vi "Find All Zeros of f(x) (Formula).vi"(6 "formula":string, 7 "accuracy":dbl=1e-08 format="%.2e", 8 "end":dbl=1.0 format="%.2f", 9 "start":dbl format="%.2f", 10 "algorithm":u16(ring) items=["Ridders", "Newton Raphson"], 11 "step type":u16(ring) items=["fixed function", "modified function"]) -> (0 "error":i32, 1 "ticks":u32, 2 "f(Zeros)":dbl[](array[numeric]) format="%.2f", 3 "Zeros":dbl[](array[numeric]) format="%.2f")   [LabVIEW 2014, in "NI_Gmath.lvlib"]
doc: "Determines all zeros of a 1D function in a given interval. You must manually select the polymorphic instance to use."
uses:
  NI_Gmath.lvlib
panel:
  # "Example:\n\n accuracy: 1E-8 \n step type: fixed function \n algorithm: Ridders \n start: 0.0\n end: 1.0\n formula: x^2+sin(x)-1"
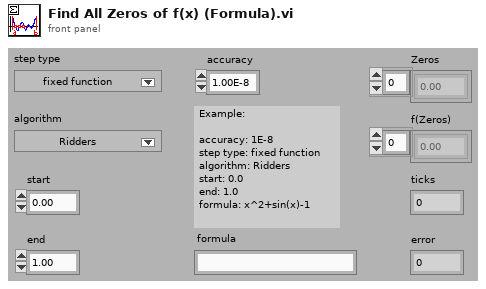
[diagram p1: front panel]
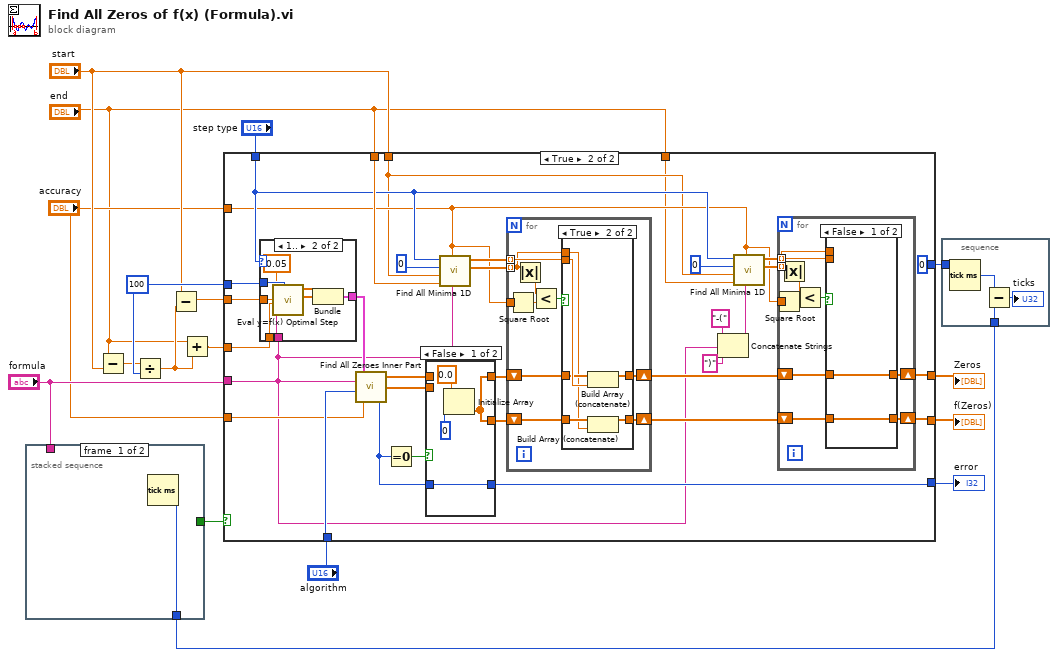
[diagram p0: block diagram]
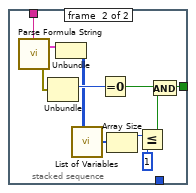
[diagram p2: hidden frame]
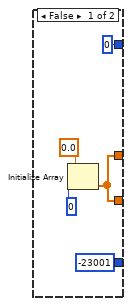
[diagram p3: hidden frame]
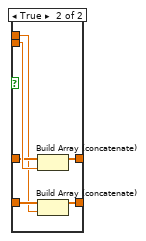
[diagram p4: hidden frame]
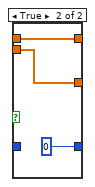
[diagram p6: hidden frame]
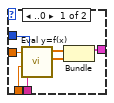
[diagram p7: hidden frame]
diagram:
  w12 = u32 100
  n1 = stacked-sequence {
    tunnel: [_ w29] -> w17
    tunnel: "formula" -> [_ w23]
    tunnel: [w18 _] -> w4
    frame #0 {
      n2 = Tick Count (ms)() -> (millisecond timer value=w18:u32)
    }
    frame #1 {
      n3 = call "Parse Formula String.vi"("formula"=w23) -> ("error out"=w22:errorcluster, "Parsed Formula"=w20:cluster{"Table":i32[][], "Y Values":dbl[]})  [unwired: 1 in]
      n4 = Unbundle(w22) -> ("code"=w21:i32)  [unwired: 2 out]
      n5 = Unbundle(w20) -> ("Table"=w19:i32[][])  [unwired: 1 out]
      n6 = call "List of Variables.vi"("Table"=w19) -> ("List of variables"=w24:i32[])
      n7 = Equal To 0?(x=w21) -> (x = 0?=w28:bool)
      n8 = Array Size(array=w24) -> (size(s)=w25:i32)
      n9 = Less Or Equal?(x=w25, y=1) -> (x <= y?=w27:bool)
      n10 = And(x=w28, y=w27) -> (x .and. y?=w29:bool)
    }
  }
  n11 = Subtract(x="end", y="start") -> (x-y=w8:dbl)
  n12 = Divide(x=w8, y=w12) -> (x/y=w7:dbl)
  n13 = Subtract(x="start", y=w7) -> (x-y=w5:dbl)
  n14 = Add(x="end", y=w7) -> (x+y=w6:dbl)
  n15 = case shown="True" w17 {
    tunnel: "step type" -> [_ w38]
    tunnel: "formula" -> [_ w40]
    tunnel: w5 -> [_ w67]
    tunnel: w6 -> [_ w66]
    tunnel: [0 0] -> w14
    tunnel: "algorithm" -> [_ w63]
    tunnel: w12 -> [_ w62]
    tunnel: [w30 w44] -> w11
    tunnel: [w30 w43] -> w10
    tunnel: [-23001 w58] -> w9
    tunnel: "accuracy" -> [_ w41]
    tunnel: "end" -> [_ w39]
    tunnel: "start" -> [_ w36]
    tunnel: "accuracy" -> [_ w37]
    tunnel: "end" -> [_ w35]
    frame False {
      n16 = Initialize Array(0.0, 0) -> (w30:dbl[])
    }
    frame True {
      n17 = case shown="1.." w38 {
        tunnel: w62 -> [w117 w122]
        tunnel: w40 -> [w114 w118]
        tunnel: w67 -> [w116 w120]
        tunnel: w66 -> [w115 w119]
        tunnel: [w111 w123] -> w64
        frame ..0 {
          n18 = call "Eval y=f(x).vi"("formula"=w114, "end"=w115, "start"=w116, "number of points"=w117) -> ("Y Values"=w112:dbl[], "X Values"=w113:dbl[])  [unwired: 2 out]
          n19 = Bundle("X Values"=w113, "Y Values"=w112) -> (w111:cluster{"X Values":dbl[], "Y Values":dbl[]})  [unwired: 1 out]
        }
        frame 1.. {
          n20 = call "Eval y=f(x) Optimal Step.vi"("number of points"=w122, "formula"=w118, "end"=w119, "start"=w120, "epsilon"=0.05) -> ("Y Values"=w124:dbl[], "X Values"=w125:dbl[])  [unwired: 2 out]
          n21 = Bundle("X Values"=w125, "Y Values"=w124) -> (w123:cluster{"X Values":dbl[], "Y Values":dbl[]})  [unwired: 1 out]
        }
      }
      n22 = call "Find All Zeroes Inner Part.vi"("accuracy"=w41, "algorithm"=w63, "formula"=w40, "X and Y values"=w64) -> ("error"=w42:i32, "f(Zeroes)"=w59:dbl[], "Zeroes"=w60:dbl[])
      n23 = Equal To 0?(x=w42) -> (x = 0?=w61:bool)
      n24 = case shown="False" w61 {
        tunnel: w60 -> [_ w110]
        tunnel: [w104 w110] -> w56
        tunnel: w59 -> [_ w109]
        tunnel: [w104 w109] -> w55
        tunnel: [w107 0] -> w58
        tunnel: w42 -> [w107 _]
        frame False {
          n25 = Initialize Array(0.0, 0) -> (w104:dbl[])
        }
        frame True {
        }
      }
      n26 = call "Find All Minima 1D.vi"("formula"=w40, "accuracy"=w37, "end"=w39, "start"=w36, "algorithm"=u16 0, "step type"=w38) -> ("f(Minima)"=w54:dbl[], "Minima"=w53:dbl[])  [unwired: 2 out]
      n27 = for {
        shift-right: [w88] -> w49
        shift-left: w56 -> [w89]
        shift-right: [w91] -> w48
        shift-left: w55 -> [w92]
        tunnel: w54 -> [w87] mode=indexing
        tunnel: w37 -> [w93]
        tunnel: w53 -> [w90] mode=indexing
        n28 = Square Root(x=w93) -> (sqrt(x)=w86:dbl)
        n29 = Absolute Value(x=w87) -> (abs(x)=w95:dbl)
        n30 = Less?(x=w95, y=w86) -> (x < y?=w94:bool)
        n31 = case shown="True" w94 {
          tunnel: w92 -> [w97 w100]
          tunnel: [w97 w99] -> w91
          tunnel: w90 -> [_ w103]
          tunnel: w89 -> [w96 w102]
          tunnel: [w96 w101] -> w88
          tunnel: w87 -> [_ w98]
          frame False {
          }
          frame True {
            n32 = Build Array (concatenate)(w102, w103) -> (w101:dbl[])
            n33 = Build Array (concatenate)(w100, w98) -> (w99:dbl[])
          }
        }
      }
      n34 = Concatenate Strings("-(", w40, ")") -> (w45:string)
      n35 = call "Find All Minima 1D.vi"("formula"=w45, "accuracy"=w37, "end"=w35, "start"=w36, "algorithm"=u16 0, "step type"=w38) -> ("f(Minima)"=w51:dbl[], "Minima"=w52:dbl[])  [unwired: 2 out]
      n36 = for {
        shift-right: [w70] -> w44
        shift-left: w49 -> [w71]
        shift-right: [w73] -> w43
        shift-left: w48 -> [w74]
        tunnel: w51 -> [w69] mode=indexing
        tunnel: w37 -> [w75]
        tunnel: w52 -> [w72] mode=indexing
        n37 = Square Root(x=w75) -> (sqrt(x)=w68:dbl)
        n38 = Absolute Value(x=w69) -> (abs(x)=w77:dbl)
        n39 = Less?(x=w77, y=w68) -> (x < y?=w76:bool)
        n40 = case shown="False" w76 {
          tunnel: w74 -> [w79 w82]
          tunnel: [w79 w81] -> w73
          tunnel: w72 -> [_ w85]
          tunnel: w71 -> [w78 w84]
          tunnel: [w78 w83] -> w70
          tunnel: w69 -> [_ w80]
          frame False {
          }
          frame True {
            n41 = Build Array (concatenate)(w84, w85) -> (w83:dbl[])
            n42 = Build Array (concatenate)(w82, w80) -> (w81:dbl[])
          }
        }
      }
    }
  }
  "Zeros" <- w11
  "f(Zeros)" <- w10
  "error" <- w9
  n43 = stacked-sequence {
    tunnel: w14 -> [_]
    tunnel: w4 -> [w126]
    frame #0 {
      n44 = Tick Count (ms)() -> (millisecond timer value=w127:u32)
      n45 = Subtract(x=w127, y=w126) -> (x-y=→"ticks":u32)
    }
  }
